vi "FTW-Publisher-Construct.vi"(5 "Address":string, 7 "Identity":string, 11 "error in":errorcluster) -> (4 "FTW-Publisher Out":refnum<class "FTW-Publisher.lvclass">, 6 "Actual Address":string, 15 "error out":errorcluster)   [LabVIEW 2013, in "FTW-Publisher.lvclass"]
uses:
  FTW-Publisher.lvclass
  Message/Base/FTW-Message.lvclass
  Listener/FTW-Listener.lvclass
  FTW-Publisher.lvclass/FTW-Publisher.ctl
  Ether/FTW-Ether.lvclass
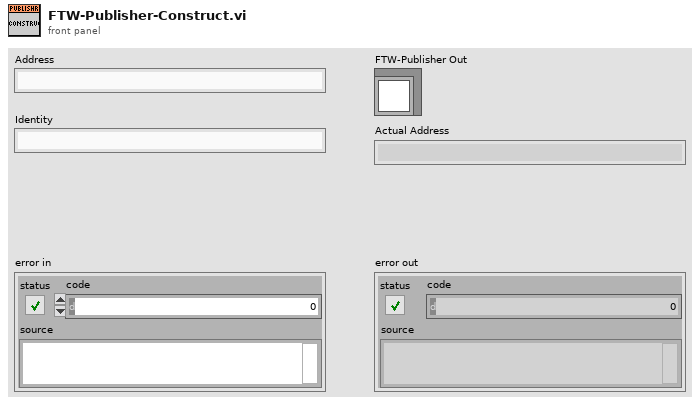
[diagram p1: front panel]
types:
  T1 = typedef "FTW-Ether.lvclass/FTW-Ether-MessageTransportScheme.ctl" = enum16{"LabVIEW Queues (lvq://)", "TCP (tcp://)", "LabVIEW Network Streams (lvns://)"}
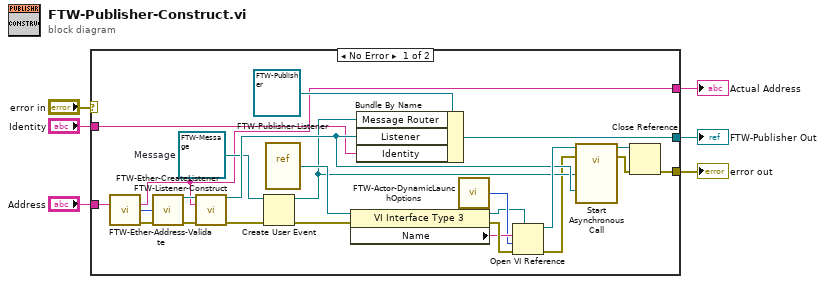
[diagram p0: block diagram]
diagram:
  n1 = case shown="No Error" "error in" {
    selector: "error in" -> [_ w31]
    tunnel: [w18 w31] -> w5
    tunnel: [w22 _] -> w4
    tunnel: "Address" -> [w14 _]
    tunnel: [w11 _] -> w2
    tunnel: "Identity" -> [w10 _]
    frame No Error {
      w15 = refnum<class "FTW-Message.lvclass"> refnum  # Message
      n2 = call "FTW-Ether-Address-Validate.vi"("Address"=w14) -> ("Sanitized Address"=w11:string, "Message Transport Scheme"=w13:T1, "error out"=w12:errorcluster)  [unwired: 12 in]
      n3 = call "FTW-Ether-CreateListener.vi"("Message Transport Scheme"=w13, "error in"=w12) -> ("FTW-Listener"=w17:refnum<class "FTW-Listener.lvclass">, "error out"=w16:errorcluster)  [unwired: 12 in]
      n4 = call-dynamic "FTW-Listener-Construct.vi"("Gmsg_Listener In"=w17, "Address"=w11, "error in"=w16) -> ("Gmsg_Listener Out"=w21:refnum<class "FTW-Listener.lvclass">, "error out"=w8:errorcluster)  [unwired: 11 in]
      n5 = Create User Event(user event datatype=w15, error in=w8) -> (user event=w20:refnum<user-event>, error out=w7:errorcluster)
      n6 = vi-ref "FTW-Publisher-Listener.vi"() -> (w30:refnum<vi>)
      n7 = property class="VI Interface Type 3"(reference=w30, error in=w7) -> (reference out=w26:refnum<vi>, error out=w29:errorcluster, "Name"=w28:string)
      n8 = Bundle By Name(cluster=refnum<class "FTW-Publisher.lvclass"> refnum ("LVmsg_Router.lvclass"), "Message Router"=w20, "Listener"=w21, "Identity"=w10) -> (w22:refnum<class "FTW-Publisher.lvclass">)
      n9 = call "FTW-Actor-DynamicLaunchOptions.vi"() -> ("Open VI Ref Options"=w27:i32)
      n10 = Open VI Reference(type specifier VI Refnum (for type only)=w26, vi path=w28, options=w27, error in (no error)=w29) -> (vi reference=w24:refnum<vi>, error out=w9:errorcluster)  [unwired: 2 in]
      n11 = call-by-ref "Start Asynchronous Call"(reference=w24, error in=w9, "Listener"=w21, "Message Publisher"=w20) -> (reference out=w19:refnum<vi>, error out=w25:errorcluster)  [unwired: 1 in]
      n12 = Close Reference(reference=w19, error in (no error)=w25) -> (error out=w18:errorcluster)
    }
    frame Error {
    }
  }
  "FTW-Publisher Out" <- w4
  "error out" <- w5
  "Actual Address" <- w2
